vi "move.vi"(8 "error in (no error)":errorcluster, 11 "FH090410SharedVariableStage in":refnum<class "StageFH090410SharedVariable.lvclass">) -> (0 "error out":errorcluster, 3 "FH090410SharedVariableStage out":refnum<class "StageFH090410SharedVariable.lvclass">)   [LabVIEW 2010, in "StageFH090410SharedVariable.lvclass"]
uses:
  StageFH090410SharedVariable.lvclass
  ControllerSimulator/space_vector_cluster.ctl
  StageDL090409Scaffold/StageDL090409Scaffold/StageDL090409Scaffold.lvclass
  StageFH090410SharedVariable.lvclass/StageFH090410SharedVariable.ctl
  common/classes/SpaceVector/SpaceVector/SpaceVector.lvclass
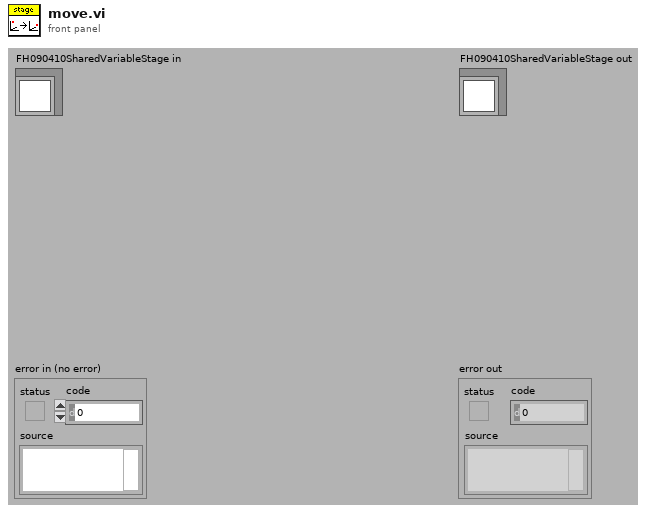
[diagram p1: front panel]
types:
  T1 = typedef "space_vector_cluster.ctl" = cluster{"x":dbl[unit], "y":dbl[unit], "z":dbl[unit]}
  T2 = typedef "StageFH090410SharedVariable.lvclass/command_mode_enum.ctl" = enum16{"step", "absolute"}
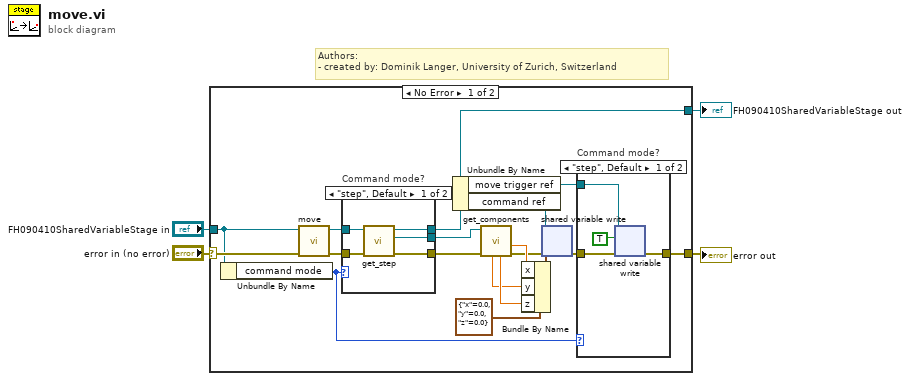
[diagram p0: block diagram]
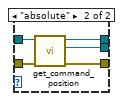
[diagram p3: hidden frame]
diagram:
  # "Authors: \n- created by: Dominik Langer, University of Zurich, Switzerland"
  n1 = case shown="No Error" "error in (no error)" {
    selector: "error in (no error)" -> [w22 w39]
    tunnel: [w12 w39] -> w3
    tunnel: [w21 w38] -> w1
    tunnel: "FH090410SharedVariableStage in" -> [w14 w38]
    frame No Error {
      n2 = Unbundle By Name(w14) -> ("command mode"=w5:T2)
      n3 = call-parent "move.vi"("error in (no error)"=w22, "DL090409StageScaffold in"=w14) -> ("error out"=w17:errorcluster, "DL090409StageScaffold out"=w16:refnum<class "StageFH090410SharedVariable.lvclass">)  [unwired: 8 out]
      n4 = case "Command mode?" shown="\"step\", Default" w5 {
        tunnel: [w29 w37] -> w21
        tunnel: [w30 w36] -> w19
        tunnel: [w28 w35] -> w18
        tunnel: w16 -> [w31 w34]
        tunnel: w17 -> [w32 w33]
        frame "step", Default {
          n5 = call-dynamic "get_step.vi"("error in (no error)"=w32, "DL090409StageScaffold in"=w31) -> ("error out"=w30:errorcluster, "step vector"=w28:refnum<class "SpaceVector.lvclass">, "DL090409StageScaffold out"=w29:refnum<class "StageFH090410SharedVariable.lvclass">)  [unwired: 7 in]
        }
        frame "absolute" {
          n6 = call-dynamic "get_command_position.vi"("error in (no error)"=w33, "DL090409StageScaffold.lvclass in"=w34) -> ("error out"=w36:errorcluster, "SpaceVector.lvclass"=w35:refnum<class "SpaceVector.lvclass">, "DL090409StageScaffold.lvclass out"=w37:refnum<class "StageFH090410SharedVariable.lvclass">)  [unwired: 7 in]
        }
      }
      n7 = Unbundle By Name(w21) -> ("move trigger ref"=w11:refnum<k21>, "command ref"=w20:refnum<k21>)
      n8 = call "get_components.vi"("error in (no error)"=w19, "SpaceVector in"=w18) -> ("error out"=w6:errorcluster, "x"=w10:dbl[unit], "z"=w9:dbl[unit], "y"=w8:dbl[unit])  [unwired: 6 out]
      n9 = Bundle By Name(cluster=T1 {"x"=0.0, "y"=0.0, "z"=0.0} ("space vector"), "x"=w10, "y"=w8, "z"=w9) -> (w7:T1)
      n10 = shared-variable-write(w20, w6, w7) -> (w13:errorcluster)  [unwired: 1 out]
      n11 = case "Command mode?" shown="\"step\", Default" w5 {
        tunnel: w13 -> [w26 w27]
        tunnel: [w25 w27] -> w12
        tunnel: w11 -> [w23 _]
        frame "step", Default {
          n12 = shared-variable-write(w23, w26, TRUE) -> (w25:errorcluster)  [unwired: 1 out]
        }
        frame "absolute" {
        }
      }
    }
    frame Error {
    }
  }
  "error out" <- w3
  "FH090410SharedVariableStage out" <- w1
